vi "backup.vi"() -> ()   [LabVIEW 2013]
panel:
  out "Waveform Chart":dbl(graph)
  in  "steps":i32
  in  "SNRs":dbl[](array[numeric])
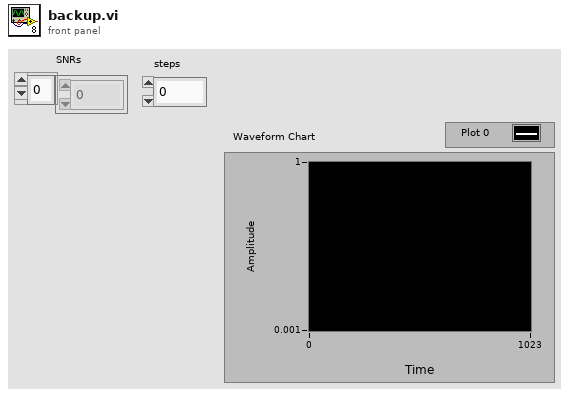
[diagram p1: front panel]
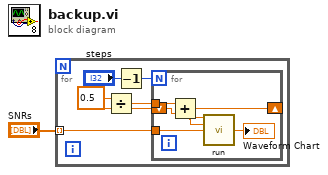
[diagram p0: block diagram]
diagram:
  n1 = for {
    tunnel: "SNRs" -> [w4] mode=indexing
    w5 = 0.5
    n2 = Divide(x=w5, y="steps") -> (x/y=w6:dbl)
    n3 = Decrement(x="steps") -> (x-1=w2:i32)
    n4 = for {
      N: w2 -> [_]
      tunnel: w6 -> [w11]
      shift-right: [w9] -> _
      shift-left: w5 -> [w10]
      tunnel: w4 -> [w8]
      n5 = Add(x=w11, y=w10) -> (x+y=w9:dbl)
      n6 = call "run.vi"("p12"=w9, "p21"=w9, "SNR"=w8) -> ("p"=→"Waveform Chart":dbl)  [unwired: 12 in]
    }
  }
